vi "Config Dual ARB Waveform.vi"(0 "VISA Resource Name":refnum<visa-resource-name>, 1 "Waveform Name (WAVEFORM)":string="WAVEFORM", 2 "Clipping Type  (0: |I + jQ|)":enum16{"|I + jQ|", "|I|, |Q|"}(ring), 3 "Clip |I| (100.0)":dbl=100.0, 4 "Clip |Q| (100.0)":dbl=100.0, 5 "error in (no error)":errorcluster {"code" format="%.0x"}, 6 "Clip |I + jQ| (100.0)":dbl=100.0, 7 "Scale (100.0)":dbl=100.0) -> (14 "VISA Resource Name Out":refnum<visa-resource-name>, 19 "error out":errorcluster {"code" format="%.0x"})   [LabVIEW 2014, in "Agilent ESG Series.lvlib"]
doc: "This VI configures Dual Arbitrary waveform adjustment.\n\nNotes:\n(1) This VI is supported for Agilent E44xxB with option UND or E4438C with option 001/601 or 002/602 only."
uses:
  Agilent ESG Series.lvlib
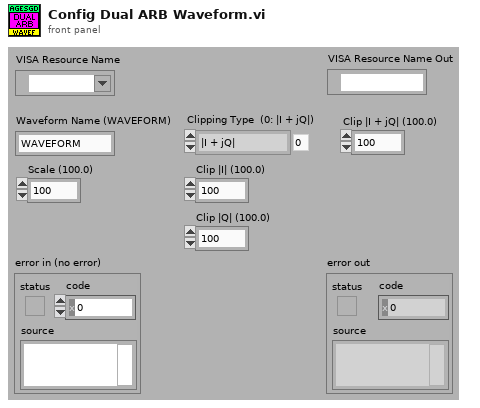
[diagram p1: front panel]
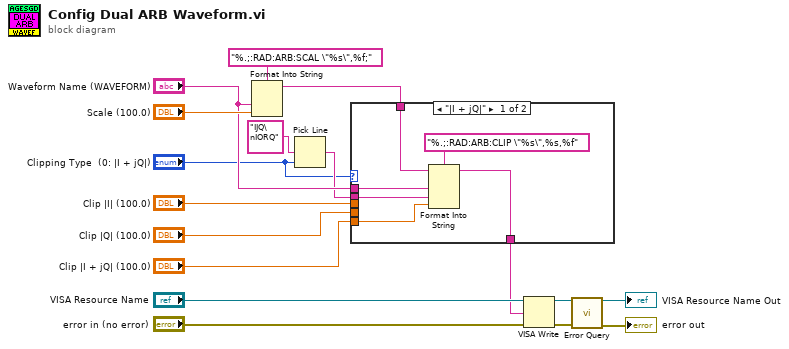
[diagram p0: block diagram]
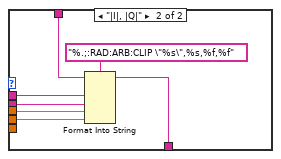
[diagram p2: hidden frame]
diagram:
  n1 = Format Into String(format string="%.;:RAD:ARB:SCAL \"%s\",%f;", "Waveform Name (WAVEFORM)", "Scale (100.0)") -> (resulting string=w3:string)  [unwired: 2 in, 1 out]
  n2 = Pick Line(multi-line string="IJQ\nIORQ", line index="Clipping Type  (0: |I + jQ|)") -> (output string=w7:string)  [unwired: 1 in]
  n3 = case shown="\"|I + jQ|\"" "Clipping Type  (0: |I + jQ|)" {
    tunnel: "Waveform Name (WAVEFORM)" -> [w22 w29]
    tunnel: w7 -> [w21 w28]
    tunnel: "Clip |I| (100.0)" -> [_ w27]
    tunnel: "Clip |Q| (100.0)" -> [_ w26]
    tunnel: "Clip |I + jQ| (100.0)" -> [w20 _]
    tunnel: w3 -> [w19 w25]
    tunnel: [w18 w24] -> w2
    frame "|I + jQ|" {
      n4 = Format Into String(format string="%.;:RAD:ARB:CLIP \"%s\",%s,%f", initial string=w19, w22, w21, w20) -> (resulting string=w18:string)  [unwired: 1 in, 1 out]
    }
    frame "|I|, |Q|" {
      n5 = Format Into String(format string="%.;:RAD:ARB:CLIP \"%s\",%s,%f,%f", initial string=w25, w29, w28, w27, w26) -> (resulting string=w24:string)  [unwired: 1 in, 1 out]
    }
  }
  n6 = VISA Write(VISA resource name="VISA Resource Name", write buffer=w2, error in (no error)="error in (no error)") -> (VISA resource name out=w13:refnum<visa-resource-name>, error out=w12:errorcluster)  [unwired: 1 out]
  n7 = call "Error Query.vi"("VISA Resource Name"=w13, "error in (no error)"=w12) -> ("VISA Resource Name Out"=→"VISA Resource Name Out":refnum<visa-resource-name>, "error out"=→"error out":errorcluster)  [unwired: 10 in, 2 out]
